vi "GetSamplingRate.vi"() -> (0 "Sampling":i32(knob) scale=0.0..10.0)   [LabVIEW 2013]
panel:
  out "Previous Time":i32=66226240
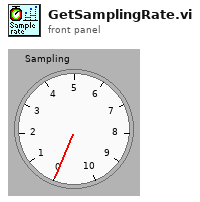
[diagram p1: front panel]
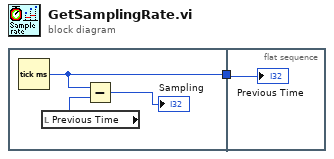
[diagram p0: block diagram]
diagram:
  n1 = flat-sequence {
    tunnel: [w3] -> w1
    tunnel: w1 -> [w5]
    frame #0 {
      n2 = Tick Count (ms)() -> (millisecond timer value=w3:u32)
      n3 = local read "Previous Time"() -> (w4:i32)
      n4 = Subtract(x=w3, y=w4) -> (x-y=→"Sampling":u32)
    }
    frame #1 {
      "Previous Time" <- w5
    }
  }
